vi "post.vi"(9 "server information":T3, 10 "application request in":T4, 11 "test responder in":refnum<class "test responder.lvclass">) -> (2 "response":T1, 3 "test responder out":refnum<class "test responder.lvclass">)   [LabVIEW 2016, in "test responder.lvclass"]
uses:
  test responder.lvclass
  HTTP server/http request.ctl
  HTTP server/http method.ctl
  HTTP headers/http header data.ctl
  HTTP server/http server info.ctl
  HTTP server/http response.ctl
  HTTP responder/https responder.lvclass
  HTTP server/Basic HTTPS server.lvclass
  HTTP headers/http headers.lvlib
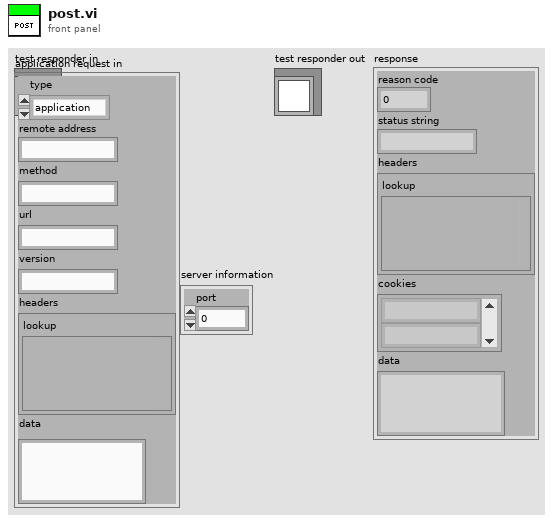
[diagram p1: front panel]
types:
  T1 = typedef "Basic HTTPS server.lvclass/http response.ctl" = cluster{"reason code":u16, "status string":string, "headers":T2, "cookies":string[], "data":string}
  T2 = typedef "http headers.lvlib/http header data.ctl" = cluster{"lookup":variant}
  T3 = typedef "Basic HTTPS server.lvclass/http server info.ctl" = cluster{"port":u16}
  T4 = typedef "Basic HTTPS server.lvclass/http request.ctl" = cluster{"type":T5, "remote address":string, "method":string, "url":string, "version":string, "headers":T2, "data":string}
  T5 = typedef "Basic HTTPS server.lvclass/http method.ctl" = enum16{"application", "error", "upgrade"}
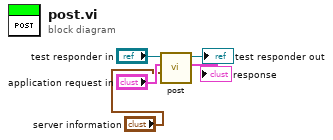
[diagram p0: block diagram]
diagram:
  n1 = call-parent "post.vi"("server information"="server information", "application request in"="application request in", "http responder in"="test responder in") -> ("response"=→"response":T1, "http responder out"=→"test responder out":refnum<class "test responder.lvclass">)  [unwired: 7 in]
